vi "Add Annotations 3.1.vi"(8 "error in":errorcluster, 10 "VI reference":refnum<vi>, 11 "File to be Annotated":path) -> (0 "error out":errorcluster, 3 "Annotated File":string)   [LabVIEW 2020]
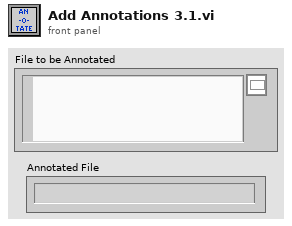
[diagram p1: front panel]
types:
  T1 = enum16{"open", "replace", "create", "open or create", "replace or create", "replace or create with confirmation"}
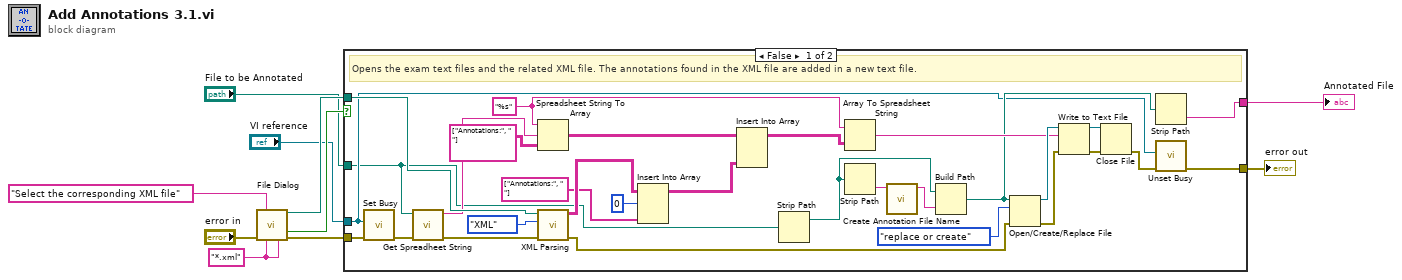
[diagram p0: block diagram]
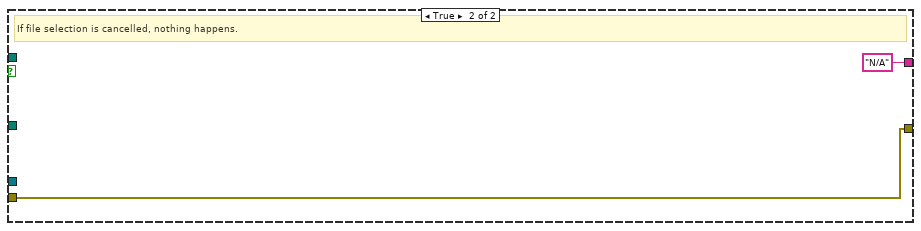
[diagram p2: hidden frame]
diagram:
  w5 = "*.xml" ("pattern label")
  n1 = call "File Dialog"("prompt"="Select the corresponding XML file", "error in"="error in", "pattern (all files)"=w5, "pattern label"=w5) -> ("selected path"=w10:path, "cancelled"=w9:bool, "error out"=w8:errorcluster)  [unwired: 8 in, 1 out]
  n2 = case shown="False" w9 {
    tunnel: w8 -> [w40 w42]
    tunnel: [w38 w42] -> w7
    tunnel: w10 -> [w21 _]
    tunnel: "File to be Annotated" -> [w11 _]
    tunnel: "VI reference" -> [w18 _]
    tunnel: [w19 "N/A" ("name")] -> w2
    frame False {
      w28 = "%s" ("format string")
      # "Opens the exam text files and the related XML file. The annotations found in the XML file are added in a new text file."
      n3 = call <vilib>:"Set Busy.vi"("error in (no error)"=w40, "VI reference (current VI)"=w18) -> ("error out"=w14:errorcluster)  [unwired: 8 in, 1 out]
      n4 = call "Get Spreadheet String.vi"("error in (no error)"=w14, "File Path"=w11) -> ("error out"=w13:errorcluster, "Spreadsheet String"=w12:string)  [unwired: 8 in]
      n5 = Spreadsheet String To Array(format string=w28, spreadsheet string=w12, array type (2D Dbl)=string[][] [["Annotations:", " "]] ("new element/subarray")) -> (array=w25:string[][])  [unwired: 1 in]
      n6 = call "XML Parsing.vi"("error in (no error)"=w13, "File Type"=enum16{"XML", "RML"}."XML", "XML File Path"=w21) -> ("error out"=w31:errorcluster, "XML Notes and Times"=w30:string[][])  [unwired: 6 in, 1 out]
      n7 = Insert Into Array "Insert Into Array"(array=w30, index (row)=0, new element=string[] ["Annotations:", " "] ("new element/subarray")) -> (w24:string[][])  [unwired: 1 in]
      n8 = Insert Into Array "Insert Into Array"(array=w25, new element=w24) -> (w23:string[][])  [unwired: 2 in]
      n9 = Strip Path(path=w11) -> (stripped path=w16:path)  [unwired: 1 out]
      n10 = Array To Spreadsheet String(array=w23, 3:w28) -> (spreadsheet string=w32:string)  [unwired: 1 in]
      n11 = Strip Path(path=w16) -> (name=w15:string)  [unwired: 1 out]
      n12 = call "Create Annotation File Name.vi"("Subject Number"=w15) -> ("File Name"=w37:string)  [unwired: 10 in]
      n13 = Build Path(base path=w16, name or relative path=w37) -> (appended path=w20:path)
      n14 = Open/Create/Replace File(file path (use dialog)=w20, error in=w31, operation (0:open)=T1."replace or create") -> (refnum out=w33:refnum<file>, error out=w17:errorcluster)  [unwired: 3 in, 1 out]
      n15 = Write to Text File(file (use dialog)=w33, text=w32, error in=w17) -> (refnum out=w34:refnum<file>, error out=w35:errorcluster)  [unwired: 1 in, 1 out]
      n16 = Close File(refnum=w34, error in=w35) -> (error out=w39:errorcluster)  [unwired: 1 out]
      n17 = Strip Path(path=w20) -> (name=w19:string)  [unwired: 1 out]
      n18 = call <vilib>:"Unset Busy.vi"("error in (no error)"=w39, "VI reference (current VI)"=w18) -> ("error out"=w38:errorcluster)  [unwired: 9 in]
    }
    frame True {
      # "If file selection is cancelled, nothing happens."
    }
  }
  "error out" <- w7
  "Annotated File" <- w2
